vi "Read (Single Response).vi"(8 "error in (no error)":errorcluster, 11 "VISA resource name":refnum<visa-resource-name>) -> (0 "error out":errorcluster, 1 "Response Bundle":T1, 2 "Response":string, 3 "VISA resource name out":refnum<visa-resource-name>)   [LabVIEW 2011, in "Zaber A Series.lvlib"]
doc: "Reads a single response from the Serial buffer. The complete string is returned on the Response output, and the details of the format of the response are described here: http://www.zaber.com/wiki/Manuals/ASCII_Protocol_Manual#Replies. This VI also parses the string, bundles the components, and returns the bundle on the Response Bundle pin. \n\nThe Response Bundle is designed to extract data from Replies only. Info and Alert type responses will not make sense in the Bundle and should be read with just the Response output. By default the only Info or Alert type responses you can expect directly follow 'help' commands. \n\nThis VI requires that the Initialize VI has been called with the same serial port. \n\nThe Data string of the response is checked for rejection responses and if any are detected will send a warning on the error out. The possible warnings are:\n\n1073481729 - BADCHECKSUM - The checksum provided in the command message was incorrect.\n1073481730 - BADCOMMAND - The command or setting is incorrect or invalid.\n1073481731 - BADDATA - The data provided in the command is incorrect or out of range.\n1073481732 - DEVICEMOVING - The device cannot be parked because it is currently moving.\n1073481733 - DEVICEONLY - An axis number was specified when trying to execute a device only command.\n1073481734 - PARKED - The device cannot move because it is currently parked.\n1073481735 - AGAIN - The stream queue is full. The command should be resent until AGAIN is not received. \n\n\nNote: This VI is set to read 100 bytes, but will terminate when it sees the new line character in order to return only one response. It's assumed that responses will be shorter than 100 characters. If your responses exceed this for any reason, adjust the constant to a higher number."
uses:
  Zaber A Series.lvlib
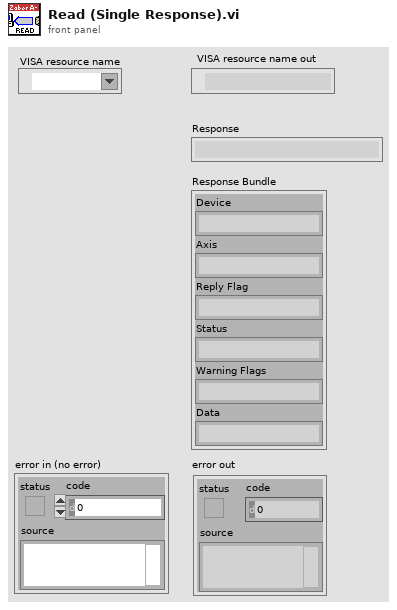
[diagram p1: front panel]
types:
  T1 = cluster{"Device":string, "Axis":string, "Reply Flag":string, "Status":string, "Warning Flags":string, "Data":string}
  T2 = cluster{"read buffer":string, "read buffer":string, "read buffer":string, "read buffer":string, "read buffer":string, "read buffer":string}
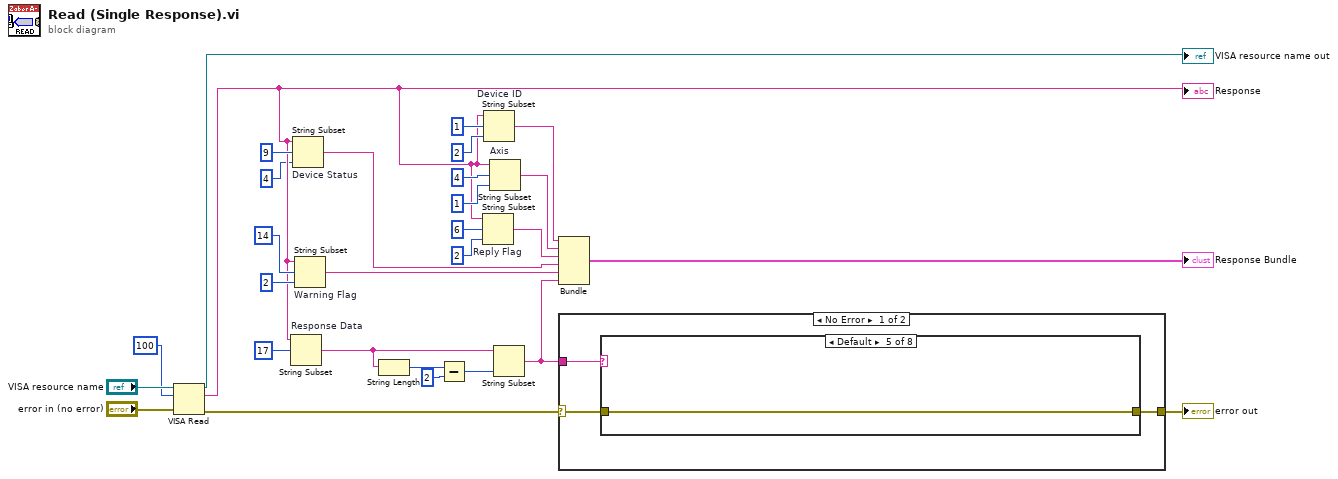
[diagram p0: block diagram]
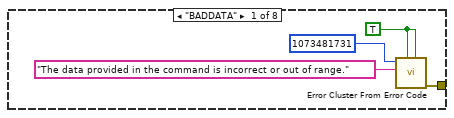
[diagram p2: hidden frame]
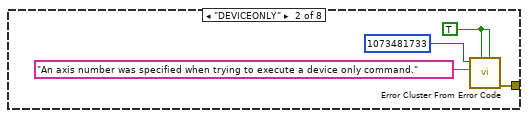
[diagram p3: hidden frame]
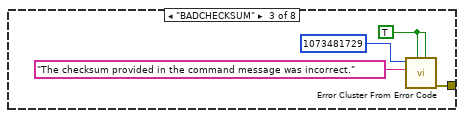
[diagram p4: hidden frame]
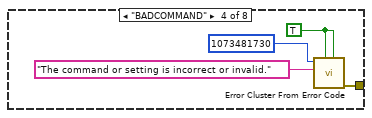
[diagram p5: hidden frame]
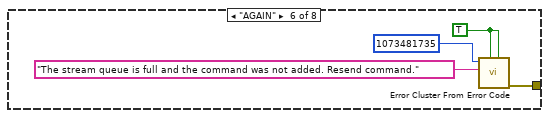
[diagram p6: hidden frame]
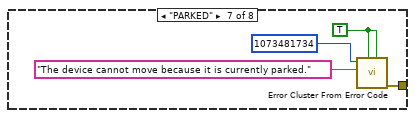
[diagram p7: hidden frame]
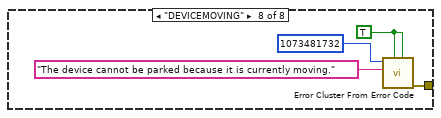
[diagram p8: hidden frame]
diagram:
  n1 = VISA Read(VISA resource name="VISA resource name", byte count=u32 100, error in (no error)="error in (no error)") -> (VISA resource name out=→"VISA resource name out":refnum<visa-resource-name>, read buffer=w5:string, error out=w4:errorcluster)  [unwired: 1 out]
  "Response" <- w5
  n2 = String Subset "Response Data"(string=w5, offset (0)=17) -> (substring=w7:string)  [unwired: 1 in]
  n3 = String Subset "Device Status"(string=w5, offset (0)=9, length (rest)=4 ("length (rest)")) -> (substring=w17:string)
  n4 = String Subset "Warning Flag"(string=w5, offset (0)=14, length (rest)=2 ("length (rest)")) -> (substring=w16:string)
  n5 = String Length(string=w7) -> (length=w10:i32)
  n6 = Subtract(x=w10, y=2) -> (x-y=w8:i32)
  n7 = String Subset "Reply Flag"(string=w5, offset (0)=6, length (rest)=2 ("length (rest)")) -> (substring=w18:string)
  n8 = String Subset "Device ID"(string=w5, offset (0)=1, length (rest)=2 ("length (rest)")) -> (substring=w15:string)
  n9 = String Subset "Axis"(string=w5, offset (0)=4, length (rest)=1 ("length (rest)")) -> (substring=w14:string)
  n10 = String Subset(string=w7, length (rest)=w8) -> (substring=w2:string)  [unwired: 1 in]
  n11 = Bundle("read buffer"=w15, "read buffer"=w14, "read buffer"=w18, "read buffer"=w17, "read buffer"=w16, "read buffer"=w2) -> (→"Response Bundle":T2)  [unwired: 1 in]
  n12 = case shown="No Error" w4 {
    selector: w4 -> [w30 w62]
    tunnel: [w32 w62] -> w3
    tunnel: w2 -> [w31 _]
    frame No Error {
      n13 = case shown="Default" w31 {
        tunnel: [w33 w39 w41 w45 w49 w50 w55 w59] -> w32
        tunnel: w30 -> [_ _ _ _ w49 _ _ _]
        frame "BADDATA" {
          w36 = TRUE
          n14 = call <vilib>:"Error Cluster From Error Code.vi"("is warning? (False)"=w36, "show call chain? (False)"=w36, "error message (\"\")"="The data provided in the command is incorrect or out of range." ("error message (\"\")"), "error code (0)"=1073481731) -> ("error out"=w33:errorcluster)  [unwired: 5 in]
        }
        frame "DEVICEONLY" {
          w40 = TRUE
          n15 = call <vilib>:"Error Cluster From Error Code.vi"("is warning? (False)"=w40, "show call chain? (False)"=w40, "error message (\"\")"="An axis number was specified when trying to execute a device only command." ("error message (\"\")"), "error code (0)"=1073481733) -> ("error out"=w39:errorcluster)  [unwired: 5 in]
        }
        frame "BADCHECKSUM" {
          w44 = TRUE
          n16 = call <vilib>:"Error Cluster From Error Code.vi"("is warning? (False)"=w44, "show call chain? (False)"=w44, "error message (\"\")"="The checksum provided in the command message was incorrect." ("error message (\"\")"), "error code (0)"=1073481729) -> ("error out"=w41:errorcluster)  [unwired: 5 in]
        }
        frame "BADCOMMAND" {
          w48 = TRUE
          n17 = call <vilib>:"Error Cluster From Error Code.vi"("is warning? (False)"=w48, "show call chain? (False)"=w48, "error message (\"\")"="The command or setting is incorrect or invalid." ("error message (\"\")"), "error code (0)"=1073481730) -> ("error out"=w45:errorcluster)  [unwired: 5 in]
        }
        frame Default {
        }
        frame "AGAIN" {
          w53 = TRUE
          n18 = call <vilib>:"Error Cluster From Error Code.vi"("is warning? (False)"=w53, "show call chain? (False)"=w53, "error message (\"\")"="The stream queue is full and the command was not added. Resend command." ("error message (\"\")"), "error code (0)"=1073481735) -> ("error out"=w50:errorcluster)  [unwired: 5 in]
        }
        frame "PARKED" {
          w57 = TRUE
          n19 = call <vilib>:"Error Cluster From Error Code.vi"("is warning? (False)"=w57, "show call chain? (False)"=w57, "error message (\"\")"="The device cannot move because it is currently parked." ("error message (\"\")"), "error code (0)"=1073481734) -> ("error out"=w55:errorcluster)  [unwired: 5 in]
        }
        frame "DEVICEMOVING" {
          w61 = TRUE
          n20 = call <vilib>:"Error Cluster From Error Code.vi"("is warning? (False)"=w61, "show call chain? (False)"=w61, "error message (\"\")"="The device cannot be parked because it is currently moving." ("error message (\"\")"), "error code (0)"=1073481732) -> ("error out"=w59:errorcluster)  [unwired: 5 in]
        }
      }
    }
    frame Error {
    }
  }
  "error out" <- w3
